vi "Turn to angle.vi"(8 "Start Time":u32, 9 "Range of accuracy":sgl, 10 "desired angle":sgl) -> (1 "In Range?":bool, 2 "coerced(x)":dbl)   [LabVIEW 2020]
doc: "turn to angle calculation in degrees"
uses:
  Robot Global Data.vi
panel:
  out "Diffrence":dbl
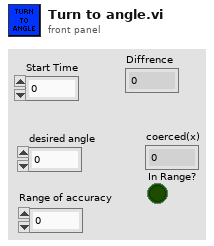
[diagram p1: front panel]
types:
  T1 = cluster{"Quat W":dbl, "Quat X":dbl, "Quat Y":dbl, "Quat Z":dbl}
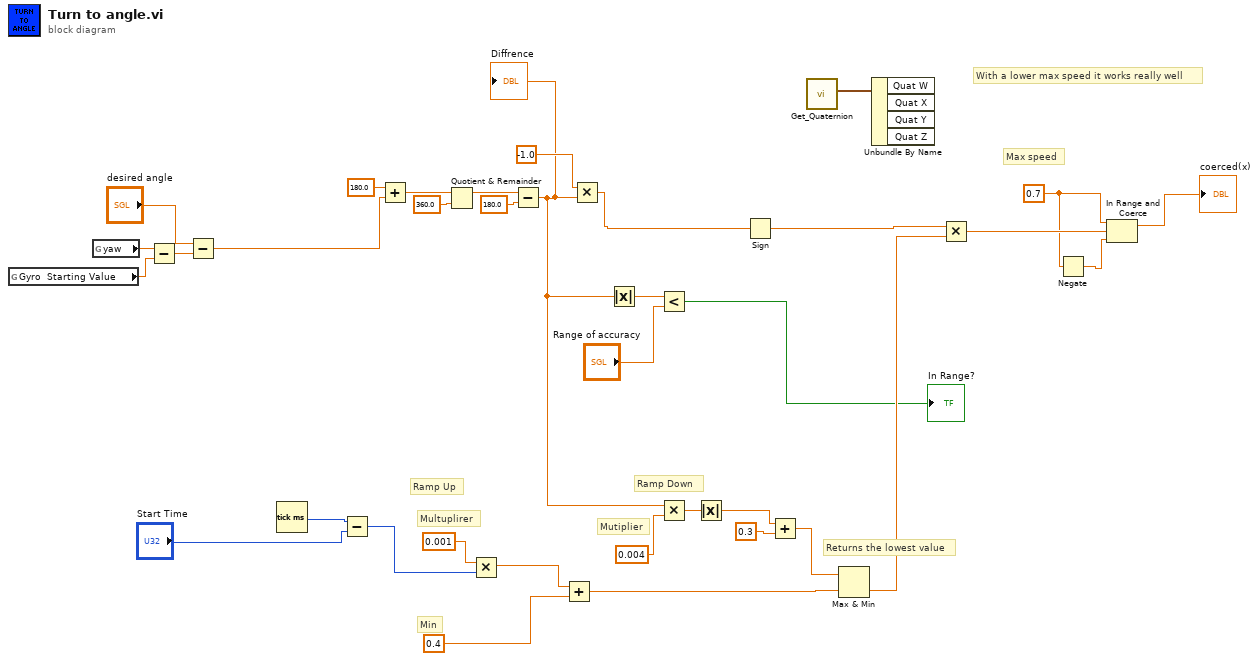
[diagram p0: block diagram]
diagram:
  w22 = 0.7 ("t")
  # "With a lower max speed it works really well"
  # "Mutiplier"
  # "Multuplirer"
  # "Min"
  # "Ramp Up"
  # "Returns the lowest value"
  # "Ramp Down"
  # "Max speed"
  n1 = global read "Robot Global Data.vi" "Gyro  Starting Value"() -> (w15:dbl)
  n2 = global read "Robot Global Data.vi" "yaw"() -> (w16:dbl)
  n3 = Subtract(x=w16, y=w15) -> (x-y=w8:dbl)
  n4 = Subtract(x="desired angle", y=w8) -> (x-y=w9:dbl)
  n5 = Tick Count (ms)() -> (millisecond timer value=w26:u32)
  n6 = Subtract(x=w26, y="Start Time") -> (x-y=w25:u32)
  n7 = Add(x=180.0, y=w9) -> (x+y=w13:dbl)
  n8 = Quotient & Remainder(x=w13, y=360.0) -> (x-y*floor(x/y)=w10:dbl)  [unwired: 1 out]
  n9 = Multiply(x=0.001 ("y"), y=w25) -> (x*y=w32:dbl)
  n10 = Subtract(x=w10, y=180.0) -> (x-y=w5:dbl)
  "Diffrence" <- w5
  n11 = Add(x=w32, y=0.4) -> (x+y=w20:dbl)
  n12 = Multiply(x=-1.0, y=w5) -> (x*y=w6:dbl)
  n13 = Absolute Value(x=w5) -> (abs(x)=w4:dbl)
  n14 = Less?(x=w4, y="Range of accuracy") -> (x < y?=→"In Range?":bool)
  n15 = Multiply(x=w5, y=0.004) -> (x*y=w30:dbl)
  n16 = Absolute Value(x=w30) -> (abs(x)=w28:dbl)
  n17 = Sign(1:w6) -> (0:w27:dbl)
  n18 = Add(x=w28, y=0.3) -> (x+y=w19:dbl)
  n19 = call <vilib>:"Get_Quaternion.vi"() -> ("Quaternion"=w1:T1)  [unwired: 11 in]
  n20 = Max & Min(x=w19, y=w20) -> (min(x,y)=w17:dbl)  [unwired: 1 out]
  n21 = Unbundle By Name(w1) -> ()  [unwired: 4 out]
  n22 = Multiply(x=w27, y=w17) -> (x*y=w23:dbl)
  n23 = Negate(x=w22) -> (-x=w21:dbl)
  n24 = In Range and Coerce(upper limit=w22, x=w23, lower limit=w21) -> (coerced(x)=→"coerced(x)":dbl)  [unwired: 1 out]
